vi "ElevatorLimitSwitchHeights.vi"(8 "error in (no error)":errorcluster) -> (0 "error out":errorcluster, 2 "LowOuter":dbl, 3 "HighOuter":dbl, 5 "LowStage3":dbl, 7 "HighStage3":dbl)   [LabVIEW 2023]
doc: "VI to set height of bottom of Elevator when limit switches are triggered\n\nInputs: none\n\nOutputs:\n--high--numeric--inches\n--low--numeric--inches"
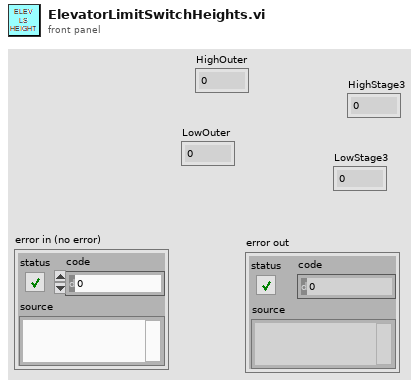
[diagram p1: front panel]
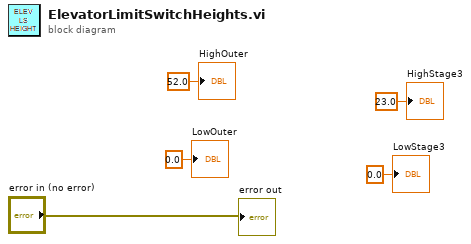
[diagram p0: block diagram]
diagram:
  "HighOuter" <- 52.0 ("high")
  "LowOuter" <- 0.0 ("low")
  "error out" <- "error in (no error)"
  "HighStage3" <- 23.0 ("HighStage3")
  "LowStage3" <- 0.0 ("LowStage3")
